vi "LEIN CMD read ACTI_6 PassThrough.vi"(7 "CMD":T1={"SID"=0, "ANF"=FALSE, "CMD"=enum."TASK", "DATA"=[]}, 11 "error in (no error)":errorcluster) -> (4 "SID":u8, 6 "Reply from sub ID":u8[](array[numeric]), 14 "ACK":bool, 15 "error out":errorcluster)   [LabVIEW 2011]
uses:
  Defenitions/LEIN CMD Cluster.ctl
  Defenitions/LEIN CMD List.ctl
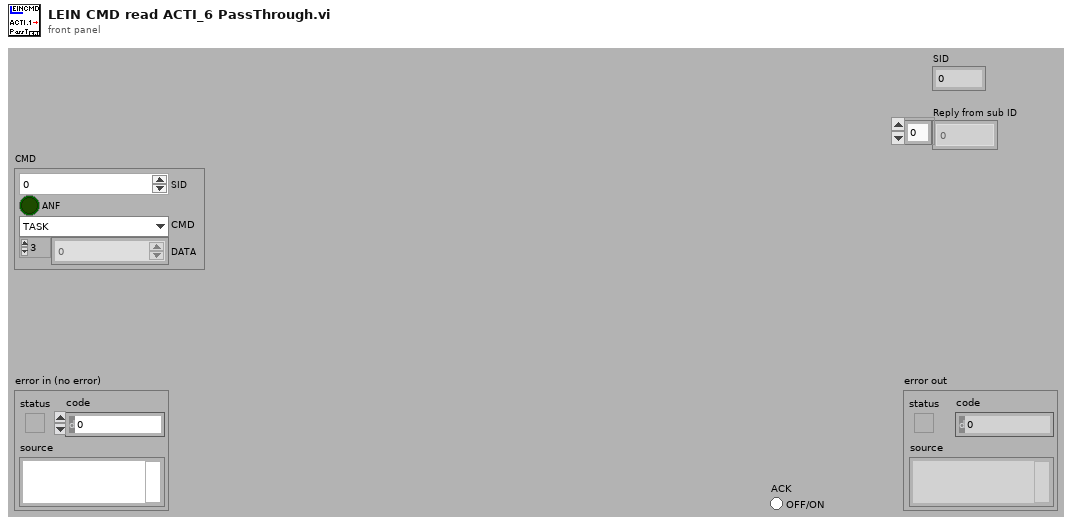
[diagram p1: front panel]
types:
  T1 = typedef "LEIN CMD Cluster.ctl" = cluster{"SID":u8, "ANF":bool, "CMD":T2, "DATA":u8[]}
  T2 = typedef "LEIN CMD List.ctl" = enum8{"ACTI", "TASK", "RES0", "STAT", "RES1", "RES2", "RES3", "USER"}
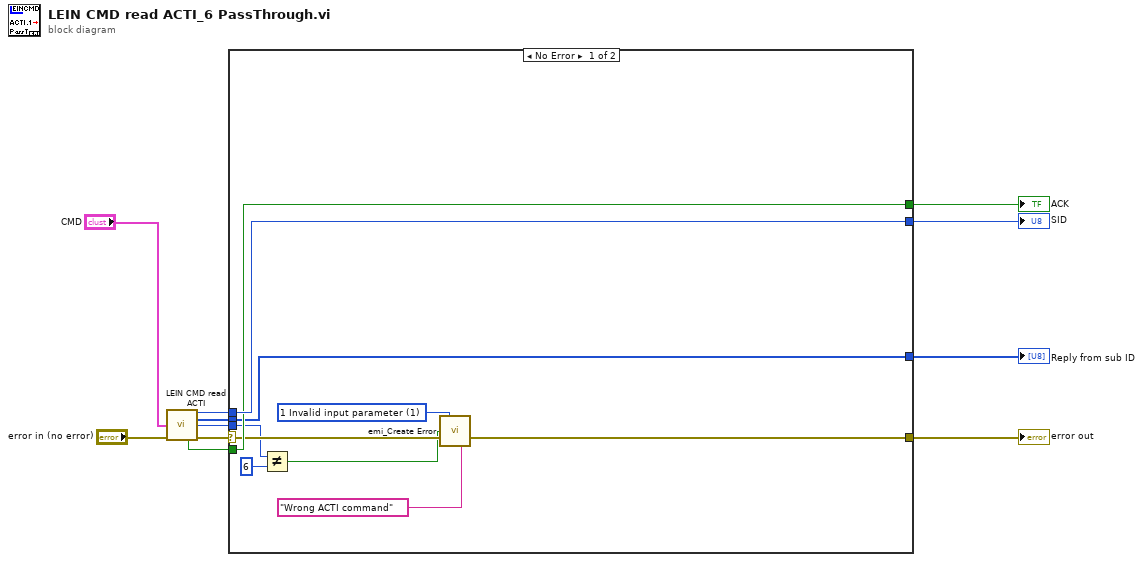
[diagram p0: block diagram]
diagram:
  n1 = call "LEIN CMD read ACTI.vi"("CMD"="CMD", "error in (no error)"="error in (no error)") -> ("SID"=w7:u8, "Data"=w8:u8[], "ACI ID"=w2:u8, "ACK"=w5:bool, "error out"=w9:errorcluster)  [unwired: 9 in]
  n2 = case shown="No Error" w9 {
    selector: w9 -> [w17 w22]
    tunnel: w8 -> [w12 _]
    tunnel: w7 -> [w21 _]
    tunnel: [w21 _] -> w6
    tunnel: w5 -> [w20 _]
    tunnel: [w20 _] -> w4
    tunnel: [w16 w22] -> w3
    tunnel: w2 -> [w15 _]
    tunnel: [w12 _] -> w1
    frame No Error {
      w19 = 1 items=["0 No Error"=0, "1 Invalid input parameter"=1, "6 Generic file IO "=6, "7 File not Found"=7, "35 Generic Pring Error"=35, "37 Device not Found"=37, "39 Device Unit Error"=39, "40 Could fot Open Device"=40, "42 Generic Error"=42, "52 Unknown Message"=52, "98 Bad File type"=98, "99 Bad File Version"=99, "100 Bad Data in File"=100, "1018 Unspecefied Error"=1018, "1041 Incorrect Password"=1041, "1043 Feature not in this version"=1043, "1109 Unsuported Data type"=1109, "1444 Did not close sucessfully"=1444] ("Error Code")
      n3 = Not Equal?(x=w15, y=u8 6) -> (x != y?=w13:bool)
      n4 = call "emi_Create Error.vi"("Error Code"=w19, "Error(T)"=w13, "error in (no error)"=w17, "Append String(\"\")"="Wrong ACTI command" ("Append String(\"\")")) -> ("error out"=w16:errorcluster)  [unwired: 11 in]
    }
    frame Error {
    }
  }
  "error out" <- w3
  "SID" <- w6
  "ACK" <- w4
  "Reply from sub ID" <- w1
